vi "EE_DataLoggingLoopXML.vi"(6 "StopButton Refnum":refnum<vi>, 8 "EEG Record Refnum":refnum<vi>, 9 "UserName":string, 10 "Logs directory path":path, 11 "ChannelsDataNotifier in":T1) -> (3 "ChannelsDataNotifier out":T1)   [LabVIEW 2016, in "Emotiv Epoc.lvlib"]
uses:
  Emotiv Epoc.lvlib
  EE_Notifier_Refnum.ctl
  EE_Notifier_Data_Type.ctl
  EE_SignalStrength_enum.ctl
  EE_EEG_ContactQuality_enum.ctl
  _XML_EEG_File_Parser/_vlib/XML_EEG_Dataset.ctl
  _XML_EEG_File_Parser/_vlib/XML_EEG_File.lvclass
  _XML_EEG_File_Parser/XML_EEG_File_Parser.lvlib
  EmotivEpocHeadsetControls.lvclass
panel:
  # "This VI is a part of BCI Design library, http://www.ru-bci.org \nCopyright © 2020, Sotnikov Peter, All rights reserved. License: CC BY-NC 4.0"
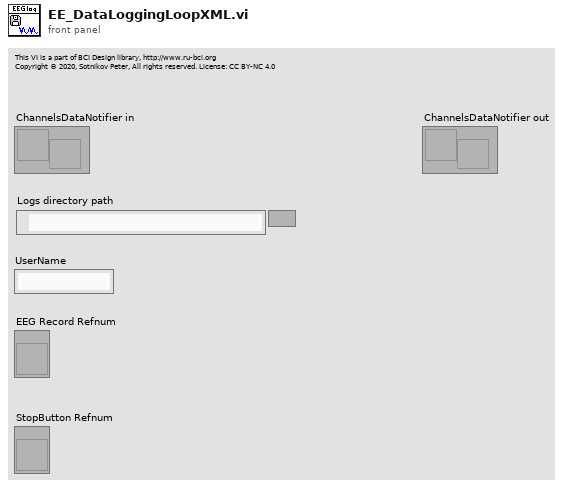
[diagram p1: front panel]
types:
  T1 = typedef "Emotiv Epoc.lvlib/EE_Notifier_Refnum.ctl" = refnum<notifier>
  T2 = typedef "XML_EEG_File_Parser.lvlib/XML_EEG_Dataset.ctl" = cluster{"Attributes":cluster{"NumberOfSamples":i32, "StartDateTime":timestamp}, "Body":cluster{"MarkerValue":string, "Channels":waveform(dbl)[]}}
  T3 = typedef "XML_EEG_File_Parser.lvlib/XML_EEG_Header.ctl" = cluster{"Attributes":cluster{"ChannelDataType":string, "NumberOfChannels":i32, "SampleRateHz":dbl, "MarkerChannel":i32}, "Body":cluster{"PatientSpecificData":string, "NumberOfDatasets":i32, "Channels":string[]}}
  T4 = typedef "Emotiv Epoc.lvlib/EE_Notifier_Data_Type.ctl" = cluster{"EDK_Error":string, "Number of samples":u32, "Marker Waveform":waveform(dbl), "Array of EEG waveforms":waveform(dbl)[], "WirelessSignalStatus":T5, "EEG_ContactsQuality":T6[]}
  T5 = typedef "Emotiv Epoc.lvlib/EmotivEpocHeadsetControls.lvclass/EE_SignalStrength_enum.ctl" = enum32{"NO_SIGNAL", "BAD_SIGNAL", "GOOD_SIGNAL"}
  T6 = typedef "Emotiv Epoc.lvlib/EE_EEG_ContactQuality_enum.ctl" = enum16{"EEG_CQ_NO_SIGNAL", "EEG_CQ_VERY_BAD", "EEG_CQ_POOR", "EEG_CQ_FAIR", "EEG_CQ_GOOD"}
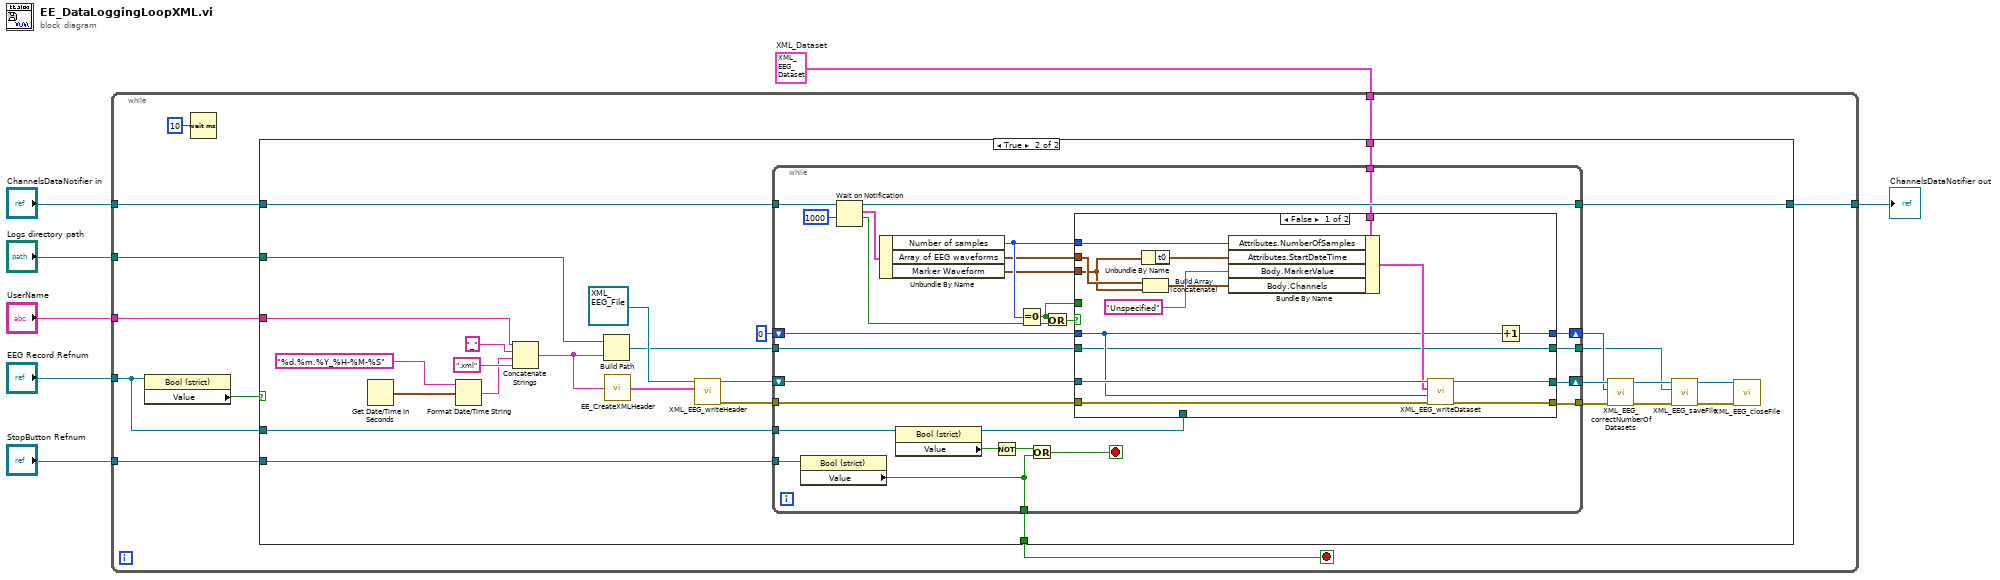
[diagram p0: block diagram]
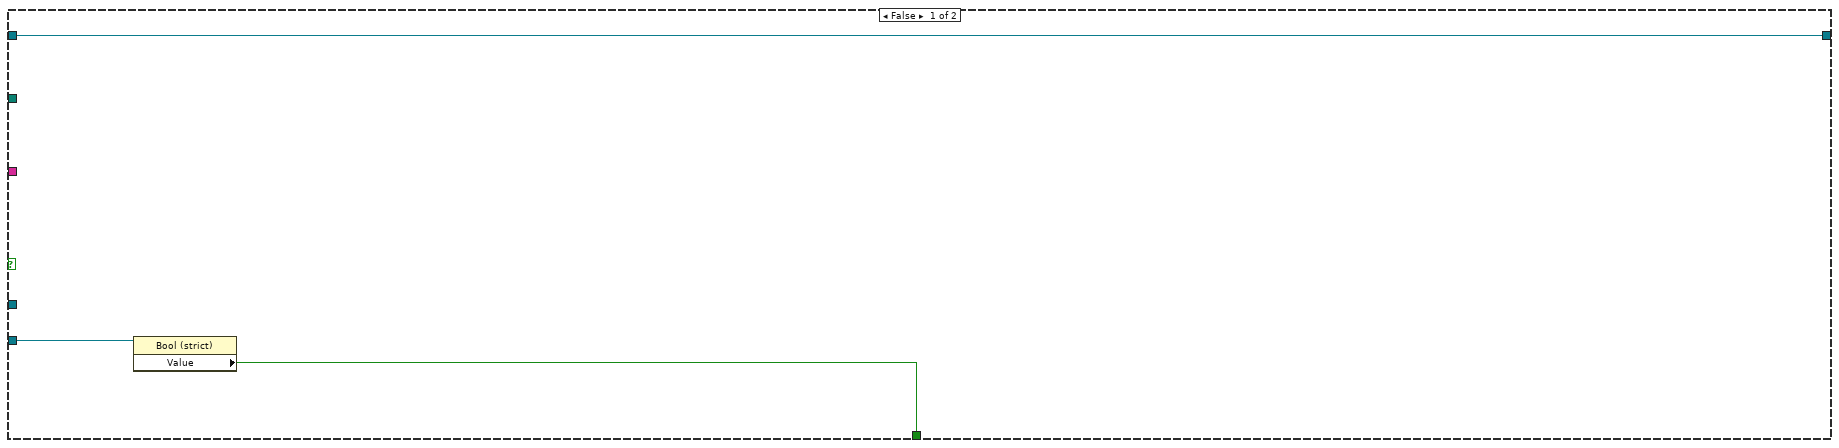
[diagram p2: hidden frame]
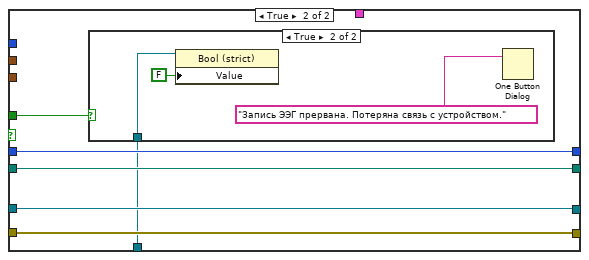
[diagram p3: hidden frame]
diagram:
  w1 = T2 {"Attributes"={"NumberOfSamples"=0, "StartDateTime"=timestamp(0 s since 1904-01-01)}, "Body"={"MarkerValue"="", "Channels"=[]}}  # XML_Dataset
  n1 = while {
    tunnel: "EEG Record Refnum" -> [w12]
    tunnel: "UserName" -> [w16]
    tunnel: "Logs directory path" -> [w15]
    tunnel: "ChannelsDataNotifier in" -> [w14]
    tunnel: [w13] -> w2
    tunnel: "StopButton Refnum" -> [w11]
    tunnel: w1 -> [w8]
    stop <- w10 stop-if-true
    n2 = property class="Bool (strict)"(reference=w12) -> ("Value"=w17:bool)  [unwired: 1 in, 2 out]
    n3 = Wait (ms)(milliseconds to wait=u32 10) -> ()  [unwired: 1 out]
    n4 = case shown="True" w17 {
      tunnel: w16 -> [_ w43]
      tunnel: w15 -> [_ w42]
      tunnel: w14 -> [w20 w41]
      tunnel: [w20 w40] -> w13
      tunnel: w12 -> [_ w39]
      tunnel: w11 -> [w19 w38]
      tunnel: [w18 w37] -> w10
      tunnel: w8 -> [_ w36]
      frame False {
        n5 = property class="Bool (strict)"(reference=w19) -> ("Value"=w18:bool)  [unwired: 1 in, 2 out]
      }
      frame True {
        n6 = Get Date/Time In Seconds() -> (seconds since 1Jan1904=w44:timestamp)
        n7 = Format Date/Time String(time format string (%c)="%d.%m.%Y_%H-%M-%S", seconds (now)=w44) -> (date/time string=w46:string)  [unwired: 1 in]
        n8 = Concatenate Strings(w43, "_" ("string"), w46, ".xml" ("string")) -> (w31:string)
        n9 = Build Path(base path=w42, name or relative path=w31) -> (appended path=w23:path)
        n10 = call "EE_CreateXMLHeader.vi"("UserName"=w31) -> ("XML_Header out"=w30:T3)  [unwired: 2 in]
        n11 = call "XML_EEG_writeHeader.vi"("XML_Header"=w30, "XML_EEG_File in"=refnum<class "XML_EEG_File.lvclass"> refnum) -> ("error out"=w21:errorcluster, "XML_EEG_File out"=w22:refnum<class "XML_EEG_File.lvclass">)  [unwired: 7 in, 1 out]
        n12 = while {
          tunnel: w23 -> [w74]
          tunnel: w41 -> [w73]
          tunnel: [w71] -> w40
          tunnel: w39 -> [w70]
          tunnel: w38 -> [w69]
          tunnel: [w65] -> w37
          tunnel: w21 -> [w64]
          tunnel: w36 -> [w62]
          shift-right: [w60] -> w32
          shift-left: 0 -> [w61]
          tunnel: [w59] -> w34
          tunnel: [w57] -> w26
          shift-right: [w58] -> w33
          shift-left: w22 -> [w63]
          stop <- w66 stop-if-true
          n13 = property class="Bool (strict)"(reference=w69) -> ("Value"=w65:bool)  [unwired: 1 in, 2 out]
          n14 = Wait on Notification(notifier=w73, timeout in ms (-1)=1000) -> (notifier out=w71:T1, notification=w56:T4, timed out?=w54:bool)  [unwired: 2 in, 1 out]
          n15 = Unbundle By Name(w56) -> ("Number of samples"=w53:u32, "Array of EEG waveforms"=w52:waveform(dbl)[], "Marker Waveform"=w51:waveform(dbl))
          n16 = property class="Bool (strict)"(reference=w70) -> (reference out=w49:refnum<vi>, "Value"=w68:bool)  [unwired: 1 in, 1 out]
          n17 = Not(x=w68) -> (.not. x?=w67:bool)
          n18 = Equal To 0?(x=w53) -> (x = 0?=w50:bool)
          n19 = Or(x=w67, y=w65) -> (x .or. y?=w66:bool)
          n20 = Or(x=w50, y=w54) -> (x .or. y?=w55:bool)
          n21 = case shown="False" w55 {
            tunnel: w74 -> [w82 w92]
            tunnel: w64 -> [w86 w93]
            tunnel: w63 -> [w87 w94]
            tunnel: w62 -> [w89 _]
            tunnel: w61 -> [w84 w95]
            tunnel: [w83 w95] -> w60
            tunnel: [w75 w93] -> w59
            tunnel: [w76 w94] -> w58
            tunnel: [w82 w92] -> w57
            tunnel: w53 -> [w81 _]
            tunnel: w52 -> [w80 _]
            tunnel: w51 -> [w79 _]
            tunnel: w50 -> [_ w91]
            tunnel: w49 -> [_ w90]
            frame False {
              n22 = Unbundle By Name(w79) -> ("t0"=w77:timestamp)
              n23 = Build Array (concatenate)(w80, w79) -> (w78:waveform(dbl)[])
              n24 = Bundle By Name(cluster=w89, "Attributes.NumberOfSamples"=w81, "Attributes.StartDateTime"=w77, "Body.MarkerValue"="Unspecified", "Body.Channels"=w78) -> (w85:T2)
              n25 = call "XML_EEG_writeDataset.vi"("error in (no error)"=w86, "DatasetNumber"=w84, "XML_Dataset"=w85, "XML_EEG_File in"=w87) -> ("error out"=w75:errorcluster, "XML_EEG_File out"=w76:refnum<class "XML_EEG_File.lvclass">)  [unwired: 5 in, 1 out]
              n26 = Increment(x=w84) -> (x+1=w83:i32)
            }
            frame True {
              n27 = case shown="True" w91 {
                tunnel: w90 -> [_ w98]
                frame False {
                }
                frame True {
                  n28 = property class="Bool (strict)"(reference=w98, "Value"=FALSE) -> ()  [unwired: 1 in, 2 out]
                  n29 = One Button Dialog(message="Запись ЭЭГ прервана. Потеряна связь с устройством.") -> ()  [unwired: 1 in, 1 out]
                }
              }
            }
          }
        }
        n30 = call "XML_EEG_correctNumberOfDatasets.vi"("error in (no error)"=w34, "NumberOfDatasets"=w32, "XML_EEG_File in"=w33) -> ("error out"=w28:errorcluster, "XML_EEG_File out"=w27:refnum<class "XML_EEG_File.lvclass">)  [unwired: 6 in, 1 out]
        n31 = call "XML_EEG_saveFile.vi"("error in (no error)"=w28, "XML file path"=w26, "XML_EEG_File in"=w27) -> ("error out"=w24:errorcluster, "XML_EEG_File out"=w25:refnum<class "XML_EEG_File.lvclass">)  [unwired: 7 in]
        n32 = call "XML_EEG_closeFile.vi"("error in (no error)"=w24, "XML_EEG_File.lvclass"=w25) -> ()  [unwired: 9 in, 1 out]
      }
    }
  }
  "ChannelsDataNotifier out" <- w2
